vi "Sprawdz Zakres Poz.vi"(8 "error in (no error)":errorcluster, 10 "Pos in":T1, 11 "Swiat Size":T2) -> (0 "error out":errorcluster, 3 "Pos out":T1)   [LabVIEW 2014, in "Swiat.lvclass"]
uses:
  Swiat.lvclass
  <vilib>/Utility/miscctls.llb/LVBoundsTypeDef.ctl
  Typedefs/Position.ctl
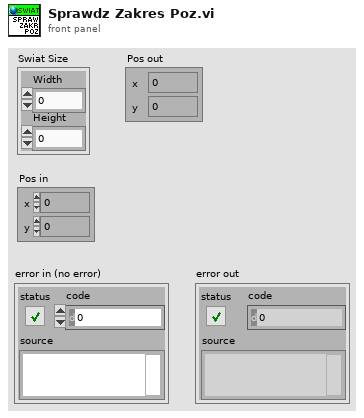
[diagram p1: front panel]
types:
  T1 = typedef "Position.ctl" = cluster{"x":i16, "y":i16}
  T2 = typedef "LVBoundsTypeDef.ctl" = cluster{"Width":u32, "Height":u32}
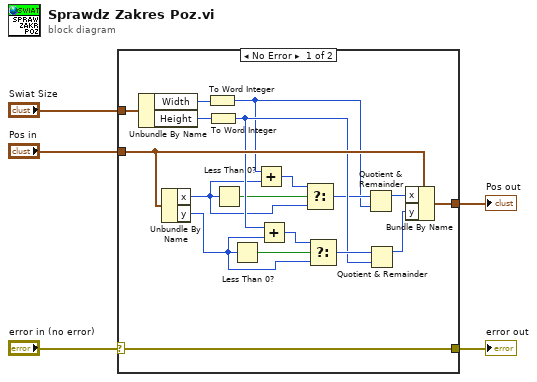
[diagram p0: block diagram]
diagram:
  n1 = case shown="No Error" "error in (no error)" {
    selector: "error in (no error)" -> [w16 w25]
    tunnel: "Swiat Size" -> [w21 _]
    tunnel: [w18 w24] -> w4
    tunnel: "Pos in" -> [w17 w24]
    tunnel: [w16 w25] -> w1
    frame No Error {
      n2 = Unbundle By Name(w21) -> ("Width"=w22:u32, "Height"=w23:u32)
      n3 = Unbundle By Name(w17) -> ("x"=w8:i16, "y"=w13:i16)
      n4 = To Word Integer(number=w22) -> (16bit integer=w6:i16)
      n5 = To Word Integer(number=w23) -> (16bit integer=w12:i16)
      n6 = Less Than 0?(x=w8) -> (x < 0?=w9:bool)
      n7 = Less Than 0?(x=w13) -> (x < 0?=w14:bool)
      n8 = Add(x=w6, y=w8) -> (x+y=w10:i16)
      n9 = Add(x=w12, y=w13) -> (x+y=w11:i16)
      n10 = Select(t=w10, s=w9, f=w8) -> (s? t:f=w7:i16)
      n11 = Select(t=w11, s=w14, f=w13) -> (s? t:f=w15:i16)
      n12 = Quotient & Remainder(x=w7, y=w6) -> (x-y*floor(x/y)=w19:i16)  [unwired: 1 out]
      n13 = Quotient & Remainder(x=w15, y=w12) -> (x-y*floor(x/y)=w20:i16)  [unwired: 1 out]
      n14 = Bundle By Name(cluster=w17, "x"=w19, "y"=w20) -> (w18:T1)
    }
    frame Error {
    }
  }
  "Pos out" <- w4
  "error out" <- w1
